vi "DSF.Engine.Framework.Initialize.Cache.vi"(8 "error in (no error)":errorcluster, 11 "Framework in":refnum<class "DSF.Engine.Framework.lvclass">) -> (0 "error out":errorcluster, 3 "Framework out":refnum<class "DSF.Engine.Framework.lvclass">)   [LabVIEW 2017, in "DSF.Engine.lvlib" / "DSF.Engine.Framework.lvclass"]
uses:
  DSF.Engine.Framework.lvclass
  DSF.Engine.Framework.lvclass/DSF.Engine.Framework.ctl
  Cache/DSF.Engine.Memory.Cache.lvclass
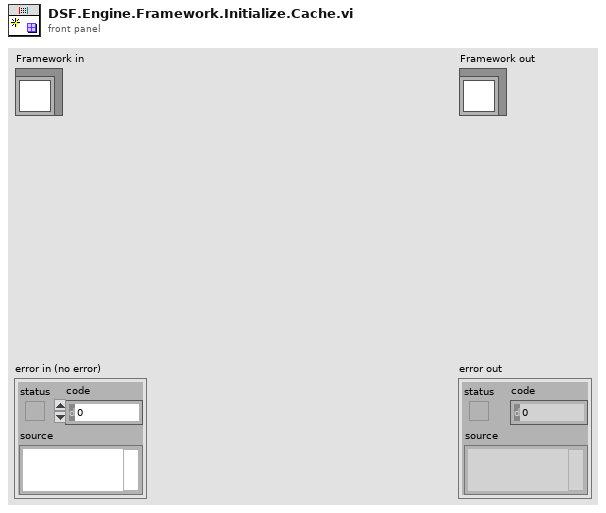
[diagram p1: front panel]
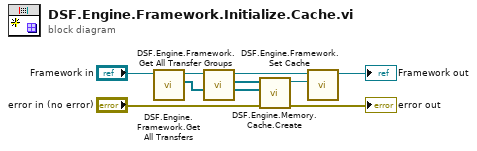
[diagram p0: block diagram]
diagram:
  n1 = call "DSF.Engine.Framework.Get All Transfers.vi"("Framework in"="Framework in") -> ("All Transfers"=w1:refnum<class "DSF.Engine.Transfer.lvclass">[], "Framework out"=w4:refnum<class "DSF.Engine.Framework.lvclass">)  [unwired: 9 in]
  n2 = call "DSF.Engine.Framework.Get All Transfer Groups.vi"("Framework in"=w4) -> ("All Transfer Groups"=w2:refnum<class "DSF.Engine.Transfer Group.lvclass">[], "Framework out"=w3:refnum<class "DSF.Engine.Framework.lvclass">)  [unwired: 9 in]
  n3 = call "DSF.Engine.Memory.Cache.Create.vi"("error in (no error)"="error in (no error)", "Transfers"=w1, "Transfers Groups"=w2) -> ("error out"=→"error out":errorcluster, "Cache out"=w9:refnum<class "DSF.Engine.Memory.Cache.lvclass">)  [unwired: 7 in]
  n4 = call "DSF.Engine.Framework.Set Cache.vi"("Cache"=w9, "Framework in"=w3) -> ("Framework out"=→"Framework out":refnum<class "DSF.Engine.Framework.lvclass">)  [unwired: 9 in]
